vi "IsControlNull.vi"(11 "CntrlRef":refnum<vi>) -> (3 "Null?":bool)   [LabVIEW 2018]
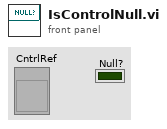
[diagram p1: front panel]
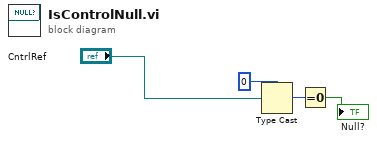
[diagram p0: block diagram]
diagram:
  n1 = Type Cast(type=0, x="CntrlRef") -> (*(type *) &x=w3:i32)
  n2 = Equal To 0?(x=w3) -> (x = 0?=→"Null?":bool)
